vi "peakdet.vi"(8 "error in":errorcluster, 9 "Delta":dbl=1.0, 10 "X":dbl[](array[numeric]), 11 "Y":dbl[](array[numeric])) -> (0 "error out":errorcluster, 1 "Peaks x,y cluster array":cluster{"X":dbl, "Y":dbl}[](array[cluster]), 2 "Valley x,y array":cluster{"X Array":dbl[], "Y array":dbl[]}, 3 "Peaks x,y arrays cluster":cluster{"X Array":dbl[], "Y array":dbl[]}, 4 "Valleys x,y cluster array":cluster{"X":dbl, "Y":dbl}[](array[cluster]), 5 "X Arr Out":dbl[](array[numeric]))   [LabVIEW 2023]
doc: "Find peaks and valleys by searching for rising signal in Y array that exceed delta value (peaks) and falling signals that exceed delta (valleys). Return arrays of peaks and valleys as arrays of x,y pair as well as clusters of x and y arrays. \n\nXout is provided in case X array input is empty. \n\nAdapted from https://billauer.co.il/blog/2009/01/peakdet-matlab-octave/"
uses:
  <vilib>/Analysis/1siggen.llb/Ramp Pattern by Delta.vi
  <vilib>/Analysis/NI_AALBase.lvlib
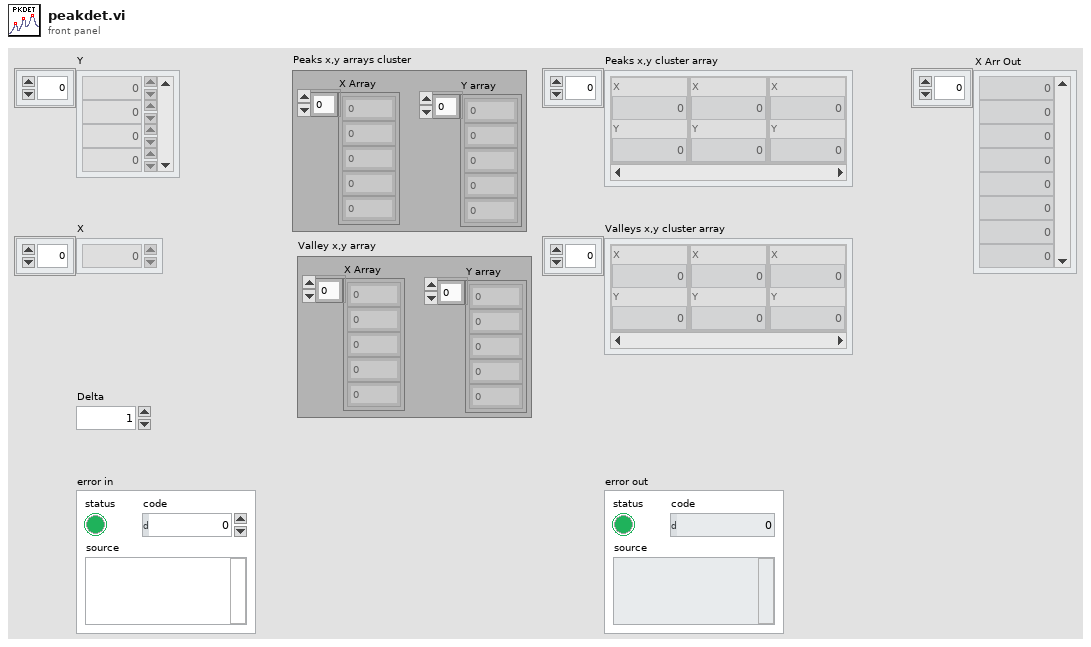
[diagram p1: front panel]
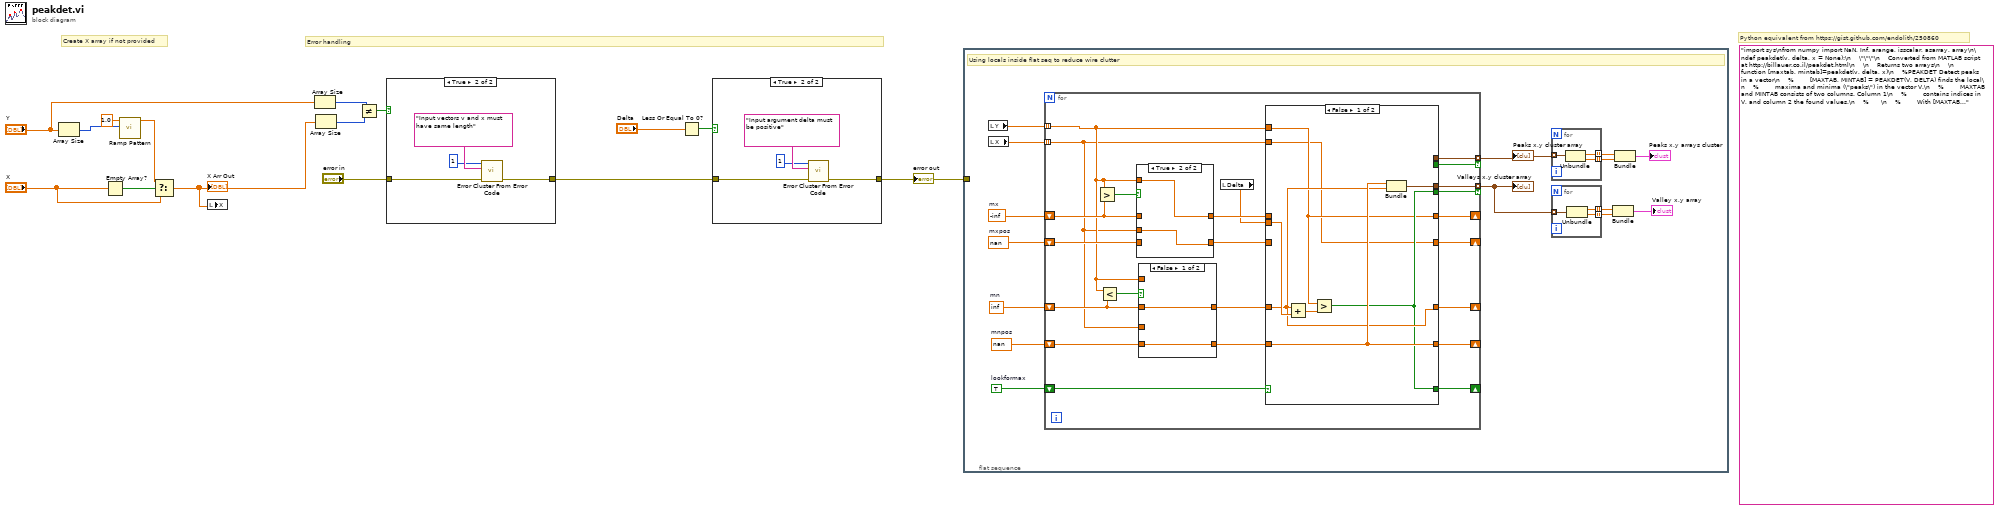
[diagram p0: block diagram]
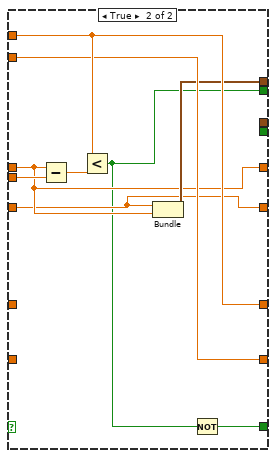
[diagram p2: hidden frame]
diagram:
  (unwired) "import sys\nfrom numpy import NaN, Inf, arange, isscalar, asarray, array\n\ndef peakdet(v, delta, x = None):\n    \"\"\"\n    Converted from MATLAB script at http://billauer.co.il/peakdet.html\n    \n    Returns two arrays\n    \n    function [maxtab, mintab]=peakdet(v, delta, x)\n    %PEAKDET Detect peaks in a vector\n    %        [MAXTAB, MINTAB] = PEAKDET(V, DELTA) finds the local\n    %        maxima and minima (\"peaks\") in the vector V.\n    %        MAXTAB and MINTAB consists of two columns. Column 1\n    %        contains indices in V, and column 2 the found values.\n    %      \n    %        With [MAXTAB, MINTAB] = PEAKDET(V, DELTA, X) the indices\n    %        in MAXTAB and MINTAB are replaced with the corresponding\n    %        X-values.\n    %\n    %        A point is considered a maximum peak if it has the maximal\n    %        value, and was preceded (to the left) by a value lower by\n    %        DELTA.\n    \n    % Eli Billauer, 3.4.05 (Explicitly not copyrighted).\n    % This function is released to the public domain; Any use is allowed.\n    \n    \"\"\"\n    maxtab = []\n    mintab = []\n       \n    if x is None:\n        x = arange(len(v))\n    \n    v = asarray(v)\n    \n    if len(v) != len(x):\n        sys.exit('Input vectors v and x must have same length')\n    \n    if not isscalar(delta):\n        sys.exit('Input argument delta must be a scalar')\n    \n    if delta <= 0:\n        sys.exit('Input argument delta must be positive')\n    \n    mn, mx = Inf, -Inf\n    mnpos, mxpos = NaN, NaN\n    \n    lookformax = True\n    \n    for i in arange(len(v)):\n        this = v[i]\n        if this > mx:\n            mx = this\n            mxpos = x[i]\n        if this < mn:\n            mn = this\n            mnpos = x[i]\n        \n        if lookformax:\n            if this < mx-delta:\n                maxtab.append((mxpos, mx))\n                mn = this\n                mnpos = x[i]\n                lookformax = False\n        else:\n            if this > mn+delta:\n                mintab.append((mnpos, mn))\n                mx = this\n                mxpos = x[i]\n                lookformax = True\n\n    return array(maxtab), array(mintab)\n\nif __name__==\"__main__\":\n    from matplotlib.pyplot import plot, scatter, show\n    series = [0,0,0,2,0,0,0,-2,0,0,0,2,0,0,0,-2,0]\n    maxtab, mintab = peakdet(series,.3)\n    plot(series)\n    scatter(array(maxtab)[:,0], array(maxtab)[:,1], color='blue')\n    scatter(array(mintab)[:,0], array(mintab)[:,1], color='red')\n    show()"
  # "Python equivalent from https://gist.github.com/endolith/250860"
  # "Error handling"
  # "Create X array if not provided"
  n1 = Array Size(array="Y") -> (size(s)=w3:i32)
  n2 = Empty Array?(array="X") -> (empty?=w15:bool)
  n3 = call-poly <vilib>:"Ramp Pattern.vi"("end"=w3, "delta"=1.0) -> ("Ramp Pattern"=w4:dbl[])  [unwired: 7 in, 2 out]
  n4 = Select(t=w4, s=w15, f="X") -> (s? t:f=w1:dbl[])
  "X Arr Out" <- w1
  n5 = local write "X"(w1) -> ()
  n6 = Array Size(array="Y") -> (size(s)=w13:i32)
  n7 = Array Size(array=w1) -> (size(s)=w12:i32)
  n8 = Not Equal?(x=w13, y=w12) -> (x != y?=w11:bool)
  n9 = case shown="True" w11 {
    tunnel: [_ w18] -> w7
    tunnel: "error in" -> [_ w16]
    frame False {
    }
    frame True {
      n10 = call <vilib>:"Error Cluster From Error Code.vi"("error in (no error)"=w16, "error message (\"\")"="Input vectors v and x must have same length" ("error message (\"\")"), "error code (0)"=1) -> ("error out"=w18:errorcluster)  [unwired: 6 in]
    }
  }
  n11 = Less Or Equal To 0?(x="Delta") -> (x <= 0?=w6:bool)
  n12 = case shown="True" w6 {
    tunnel: [_ w22] -> w5
    tunnel: w7 -> [_ w20]
    frame False {
    }
    frame True {
      n13 = call <vilib>:"Error Cluster From Error Code.vi"("error in (no error)"=w20, "error message (\"\")"="Input argument delta must be positive" ("error message (\"\")"), "error code (0)"=1) -> ("error out"=w22:errorcluster)  [unwired: 6 in]
    }
  }
  "error out" <- w5
  n14 = flat-sequence {
    tunnel: w5 -> [_]
    frame #0 {
      w36 = nan  # mxpos
      w33 = nan  # mnpos
      w37 = -inf  # mx
      w34 = inf  # mn
      w32 = TRUE  # lookformax
      # "Using locals inside flat seq to reduce wire clutter"
      n15 = local read "Y"() -> (w38:dbl[])
      n16 = local read "X"() -> (w35:dbl[])
      n17 = for {
        tunnel: w38 -> [w59] mode=indexing
        shift-right: [w49] -> _
        shift-left: w37 -> [w66]
        shift-right: [w48] -> _
        shift-left: w36 -> [w65]
        tunnel: w35 -> [w56] mode=indexing
        shift-right: [w58] -> _
        shift-left: w34 -> [w63]
        shift-right: [w55] -> _
        shift-left: w33 -> [w62]
        shift-right: [w45] -> _
        shift-left: w32 -> [w53]
        tunnel: [w51] -> w31 mode=indexing if=w50
        tunnel: [w47] -> w24 mode=indexing if=w46
        n18 = Greater?(x=w59, y=w66) -> (0:w67:bool)
        n19 = Less?(x=w59, y=w63) -> (x < y?=w64:bool)
        n20 = case shown="True" w67 {
          tunnel: [w90 w92] -> w61
          tunnel: w59 -> [_ w92]
          tunnel: w66 -> [w90 _]
          tunnel: w65 -> [w89 _]
          tunnel: w56 -> [_ w91]
          tunnel: [w89 w91] -> w52
          frame False {
          }
          frame True {
          }
        }
        n21 = case shown="False" w64 {
          tunnel: w59 -> [_ w88]
          tunnel: [w86 w88] -> w57
          tunnel: w63 -> [w86 _]
          tunnel: w62 -> [w85 _]
          tunnel: [w85 w87] -> w54
          tunnel: w56 -> [_ w87]
          frame False {
          }
          frame True {
          }
        }
        n22 = local read "Delta"() -> (w60:dbl)
        n23 = case shown="False" w53 {
          tunnel: w61 -> [_ w79]
          tunnel: w60 -> [w75 w84]
          tunnel: w59 -> [w69 w82]
          tunnel: [w71 w82] -> w58
          tunnel: w57 -> [w71 _]
          tunnel: [w73 w81] -> w55
          tunnel: w56 -> [w68 w81]
          tunnel: w54 -> [w73 _]
          tunnel: w52 -> [_ w78]
          tunnel: [_ w80] -> w51
          tunnel: [_ w76] -> w50
          tunnel: [w69 w79] -> w49
          tunnel: [w68 w78] -> w48
          tunnel: [w72 _] -> w47
          tunnel: [w70 _] -> w46
          tunnel: [w70 w77] -> w45
          frame False {
            n24 = Add(x=w71, y=w75) -> (x+y=w74:dbl)
            n25 = Greater?(x=w69, y=w74) -> (0:w70:bool)
            n26 = Bundle("Y"=w73, "Y"=w71) -> (w72:cluster{"Y":dbl, "Y":dbl})  [unwired: 1 in]
          }
          frame True {
            n27 = Subtract(x=w79, y=w84) -> (x-y=w83:dbl)
            n28 = Less?(x=w82, y=w83) -> (x < y?=w76:bool)
            n29 = Bundle("Y"=w78, "Y"=w79) -> (w80:cluster{"Y":dbl, "Y":dbl})  [unwired: 1 in]
            n30 = Not(x=w76) -> (.not. x?=w77:bool)
          }
        }
      }
      "Peaks x,y cluster array" <- w31
      "Valleys x,y cluster array" <- w24
      n31 = for {
        tunnel: w31 -> [w44] mode=indexing
        tunnel: [w43] -> w30 mode=indexing
        tunnel: [w42] -> w29 mode=indexing
        n32 = Unbundle(w44) -> ("Y"=w43:dbl, "Y"=w42:dbl)
      }
      n33 = for {
        tunnel: w24 -> [w41] mode=indexing
        tunnel: [w40] -> w27 mode=indexing
        tunnel: [w39] -> w26 mode=indexing
        n34 = Unbundle(w41) -> ("Y"=w40:dbl, "Y"=w39:dbl)
      }
      n35 = Bundle(w27, w26) -> (→"Valley x,y array":cluster{dbl[], dbl[]})  [unwired: 1 in]
      n36 = Bundle(w30, w29) -> (→"Peaks x,y arrays cluster":cluster{dbl[], dbl[]})  [unwired: 1 in]
    }
  }
